vi "XIPIN_Image_Characterization_1_1.vi"   [LabVIEW 2017]
doc: "The Xilinx Image Characterization LogiCORE calculates important statistical data for video input streams. Characterization is an important processing block for many applications including face recognition, object detection, and more. Statistics include means and variances for luminance, chrominance, high and low frequencies, edges and motion (When used with the Xilinx Motion Adaptive Noise Reduction LogiCORE) on both a global and block basis. Support for block sizes of 4x4, 8x8, 16x16, 32x32 or 64x64 pixels. Support for 8-bit pixel data in YUV 4:2:2 or 4:2:0, up to 1080p 30fps. The core is programmable through a comprehensive register interface for setting edge gains, high-pass gain, color selects (hue and saturation) and block size. The Image Characterization LogiCORE is provided with two different interfaces: General purpose processor and EDK pCore (including device driver).\n------------------------------------\n<b>Need License</b> : Yes"
uses:
  <vilib>/rvi/XilinxIP/XIPIN_XNode/niFpgaXIPIN.xnode
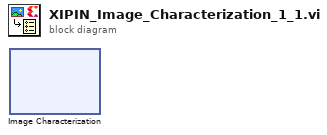
[diagram p0: block diagram]
diagram:
  n1 = xnode ("Image Characterization")() -> ()
